vi "Nov_24.vi"() -> ()   [LabVIEW 2020]
panel:
  out "?":dynamicdata(graph)
  out "?":dynamicdata(graph)
  out "?":dynamicdata(graph)
  in  "Motor Trottle":dbl(slide) scale=0.0..5.0
  out "Selected Signals":dynamicdata(graph)
  out "Signal Filtered":dynamicdata(graph)
  out "Motor":bool
  in  "Motor Enable":bool
  out "Swing":bool
  out "Hit 1":bool
  in  "Record Signal":bool
  in  "STOP":bool
  # "Gait Events"
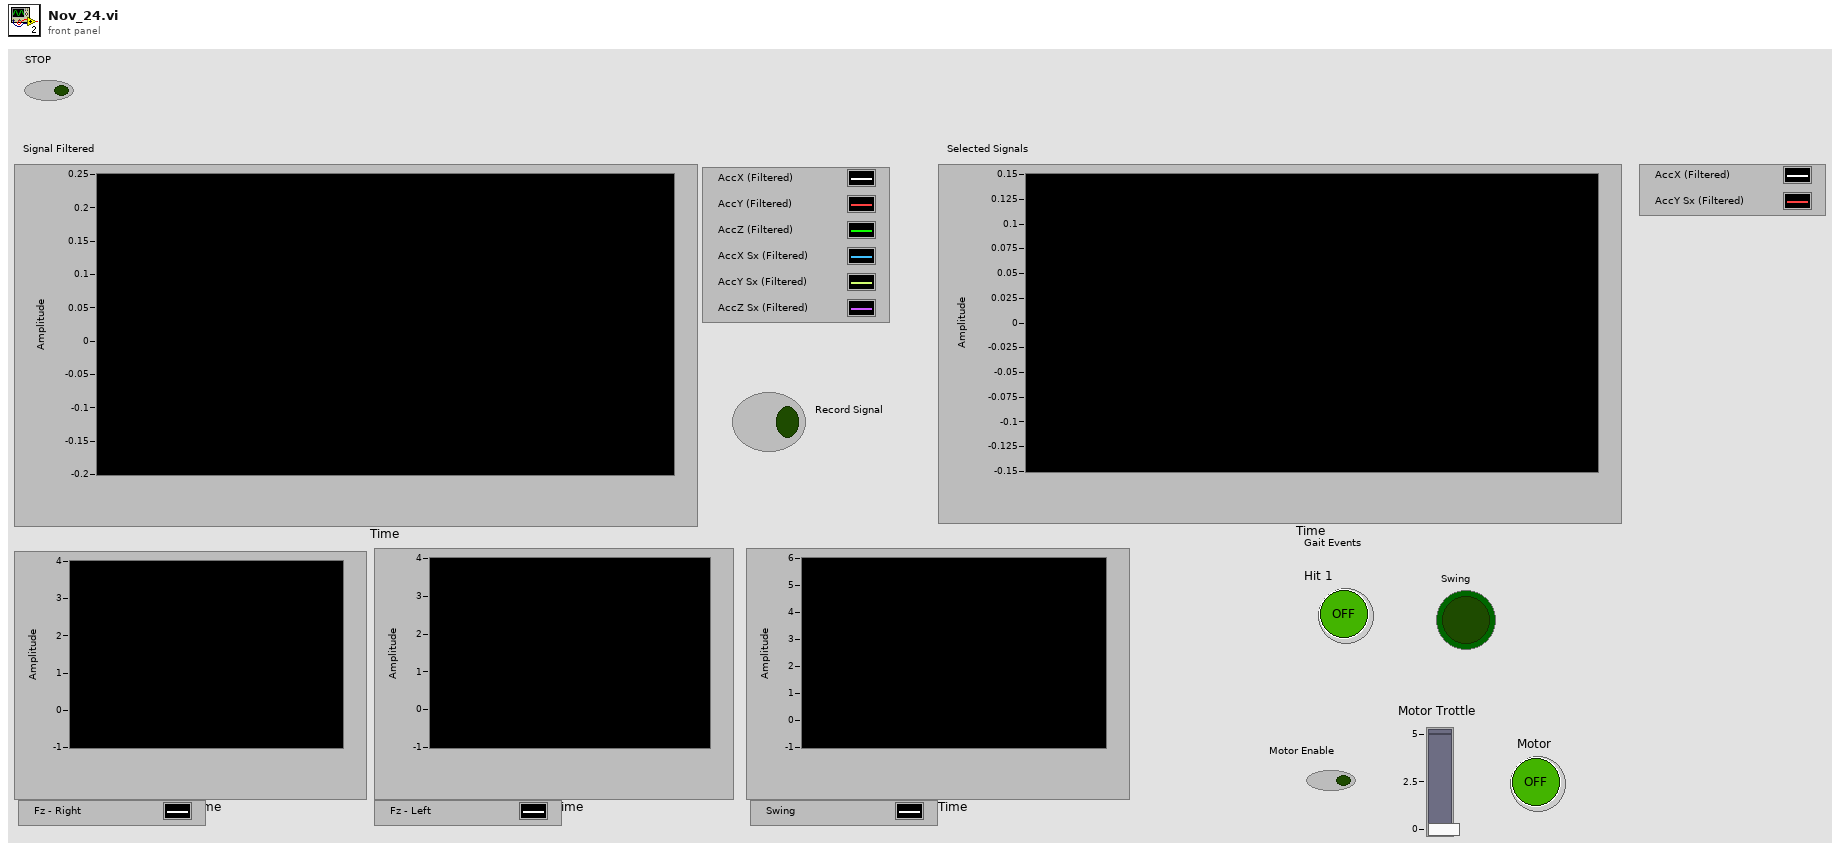
[diagram p1: front panel]
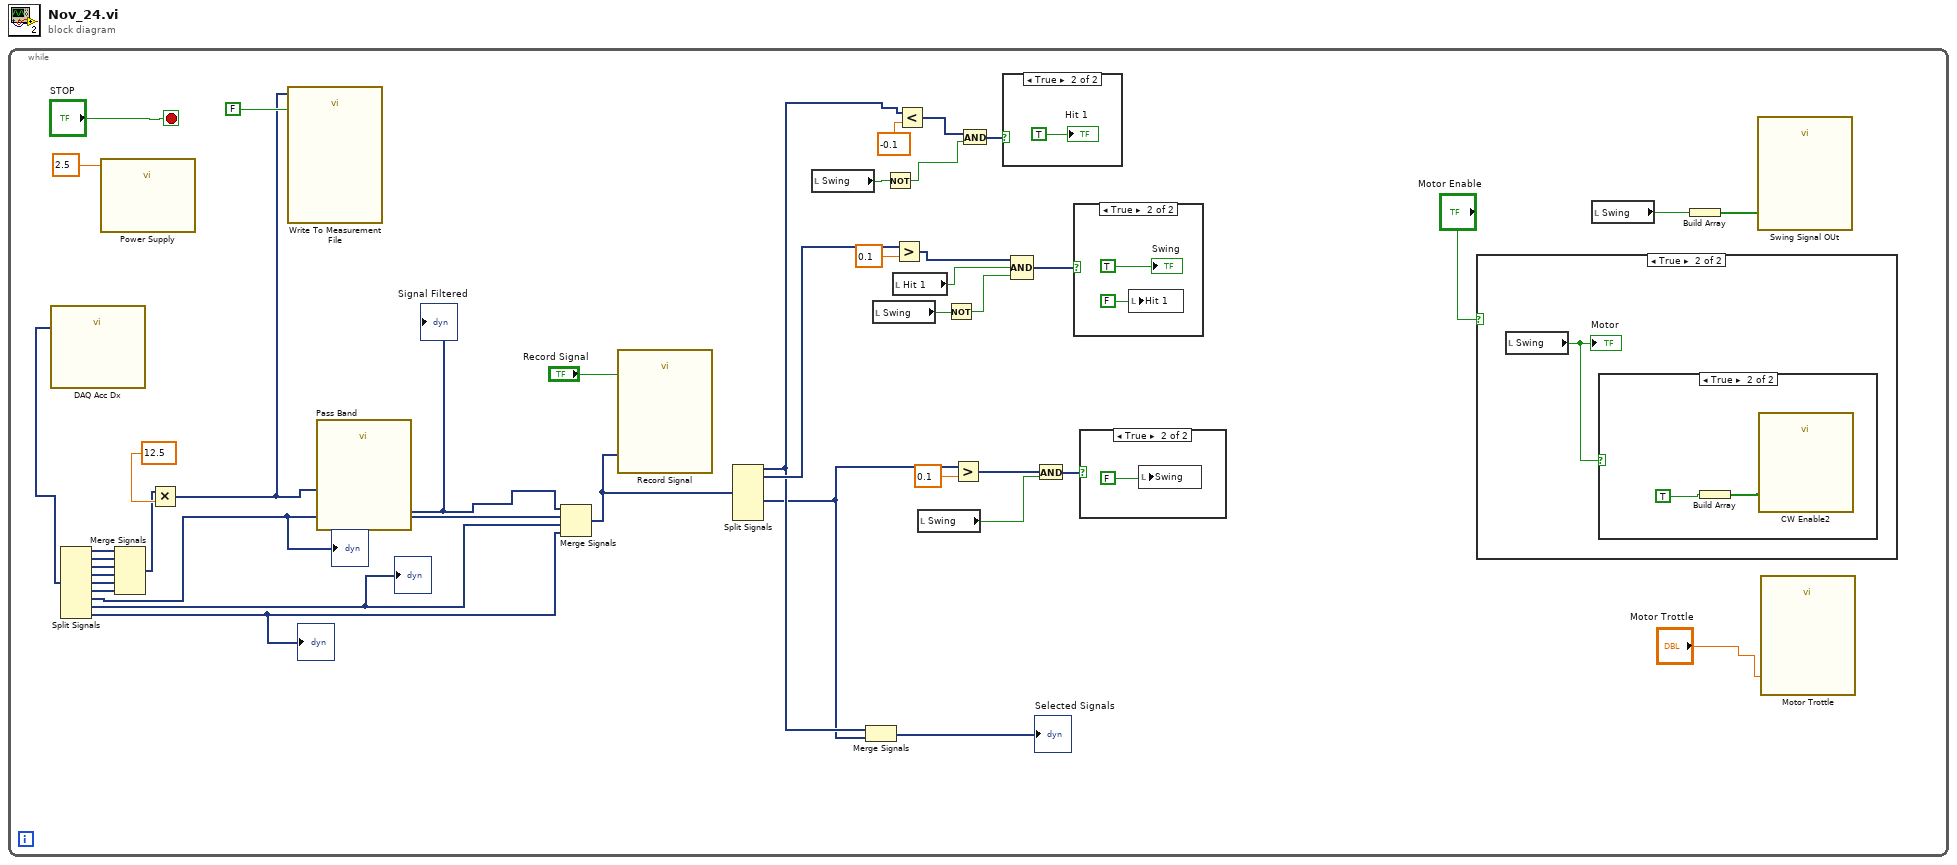
[diagram p0: block diagram]
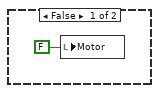
[diagram p3: hidden frame]
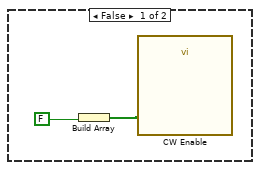
[diagram p4: hidden frame]
diagram:
  n1 = while {
    stop <- "STOP" stop-if-true
    n2 = call "DAQ Acc Dx"() -> ("data"=w29:dynamicdata)  [unwired: 16 in, 3 out]
    n3 = Split Signals(w29) -> (w28:dynamicdata, w27:dynamicdata, w26:dynamicdata, w25:dynamicdata, w24:dynamicdata, w23:dynamicdata, w21:dynamicdata, w20:dynamicdata, w19:dynamicdata)  [unwired: 9 in]
    "?" <- w21
    "?" <- w20
    "?" <- w19
    n4 = call "Power Supply"("data"=2.5) -> ()  [unwired: 17 in, 2 out]
    n5 = Merge Signals(w28, w27, w26, w25, w24, w23) -> (w22:dynamicdata)
    n6 = Multiply(x=w22, y=12.5) -> (x*y=w30:dynamicdata)
    n7 = call "Write To Measurement File"("Signals"=w30, "Enable"=FALSE) -> ()  [unwired: 15 in, 3 out]
    n8 = call "Pass Band"("Signal"=w30) -> ("Filtered Signal"=w33:dynamicdata)  [unwired: 9 in, 1 out]
    "Signal Filtered" <- w33
    n9 = Merge Signals(w33, w21, w20, w19) -> (w32:dynamicdata)
    n10 = call "Record Signal"("Signals"=w32, "Enable"="Record Signal") -> ()  [unwired: 15 in, 3 out]
    n11 = Split Signals(w32) -> (w12:dynamicdata, w15:dynamicdata, w5:dynamicdata)  [unwired: 7 in, 4 out]
    n12 = local read "Swing"() -> (w18:bool)
    n13 = Merge Signals(w12, w5) -> (→"Selected Signals":dynamicdata)
    n14 = local read "Swing"() -> (w8:bool)
    n15 = Not(x=w18) -> (.not. x?=w17:bool)
    n16 = local read "Hit 1"() -> (w10:bool)
    n17 = Greater?(x=w15, y=0.1) -> (0:w9:dynamicdata)
    n18 = Less?(x=w12, y=-0.1) -> (x < y?=w11:dynamicdata)
    n19 = local read "Swing"() -> (w2:bool)
    n20 = Not(x=w8) -> (.not. x?=w7:bool)
    n21 = Greater?(x=w5, y=0.1) -> (0:w1:dynamicdata)
    n22 = And(x=w11, y=w17) -> (x .and. y?=w16:dynamicdata)
    n23 = case shown="True" w16 {
      frame False {
      }
      frame True {
        "Hit 1" <- TRUE
      }
    }
    n24 = Compound Arithmetic op=AND(w9, w10, w7) -> (w6:dynamicdata)
    n25 = And(x=w1, y=w2) -> (x .and. y?=w3:dynamicdata)
    n26 = case shown="True" w6 {
      frame False {
      }
      frame True {
        n27 = local write "Hit 1"(FALSE) -> ()
        "Swing" <- TRUE
      }
    }
    n28 = case shown="True" w3 {
      frame False {
      }
      frame True {
        n29 = local write "Swing"(FALSE) -> ()
      }
    }
    n30 = case shown="True" "Motor Enable" {
      frame False {
        n31 = local write "Motor"(FALSE) -> ()
      }
      frame True {
        n32 = local read "Swing"() -> (w46:bool)
        "Motor" <- w46
        n33 = case shown="True" w46 {
          frame False {
            n34 = Build Array(FALSE) -> (w48:bool[])
            n35 = call "CW Enable"("data"=w48) -> ()  [unwired: 17 in, 2 out]
          }
          frame True {
            n36 = Build Array "Build Array"(TRUE) -> (w49:bool[])
            n37 = call "CW Enable2"("data"=w49) -> ()  [unwired: 17 in, 2 out]
          }
        }
      }
    }
    n38 = local read "Swing"() -> (w35:bool)
    n39 = Build Array "Build Array"(w35) -> (w34:bool[])
    n40 = call "Swing Signal OUt"("data"=w34) -> ()  [unwired: 17 in, 2 out]
    n41 = call "Motor Trottle"("data"="Motor Trottle") -> ()  [unwired: 17 in, 2 out]
  }
